vi "Alpha Ver 2.1.vi"() -> ()   [LabVIEW 2015]
uses:
  <instrlib>/Keithley 622x LV 2009/Utility/Typedefs/KE622x -- Instrument Type.ctl
  <instrlib>/Keithley 622x LV 2009/Keithley 622x.lvlib
panel:
  out "Measurements":string
  in  "Comments":string
  out "FILE":refnum<file>
  in  "Folder \nPrename":string
  out "Output command string":string
  out "Example of commands":string="*RST\nSOUR:PDEL:HIGH 1e-3\nSOUR:PDEL:LOW 0\nSOUR:PDEL:WIDT 500e-6\nSOUR:PDEL:SDEL 100e-6\nSOUR:PDEL:COUN INF\nSOUR:PDEL:RANG BEST\nSOUR:PDEL:INT 5\nSOUR:PDEL:LME 2\nTRAC:POIN 200\nSOUR:PDEL:ARM\nINIT:IMM"
  out "LM_com":string
  out "I_com":string
  out "R_com":string
  out "C_com":string
  out "SD_com":string
  out "W_com":string
  out "LL_com":string
  out "HL_com":string
  in  "INF Button":bool
  in  "prefix 2":u16(ring)
  in  "prefix":u16(ring)
  in  "Low Measure":u16(ring)=1 items=["1", "2"]
  in  "Interval":dbl=5.0 min=5.0 max=999999.0 step=1.0
  in  "Ranging":string(combo)="BEST"
  in  "Count":dbl=1.0 min=1.0 max=65536.0 step=1.0
  in  "Source Delay":dbl
  in  "Width":dbl
  in  "Low Level":dbl min=-0.105 max=0.105
  in  "High Level":dbl
  out "2182A \nconnected ?":string
  in  "STOP":bool
  out "Measurement\nUnits":string
  out "2182A Voltage \nRange":string
  out "error out":errorcluster
  # "Pulse Measurement System"
  # "SYSTEM INFORMATION"
  # "FILE CONFIGURATION"
  # "PULSE SETTINGS"
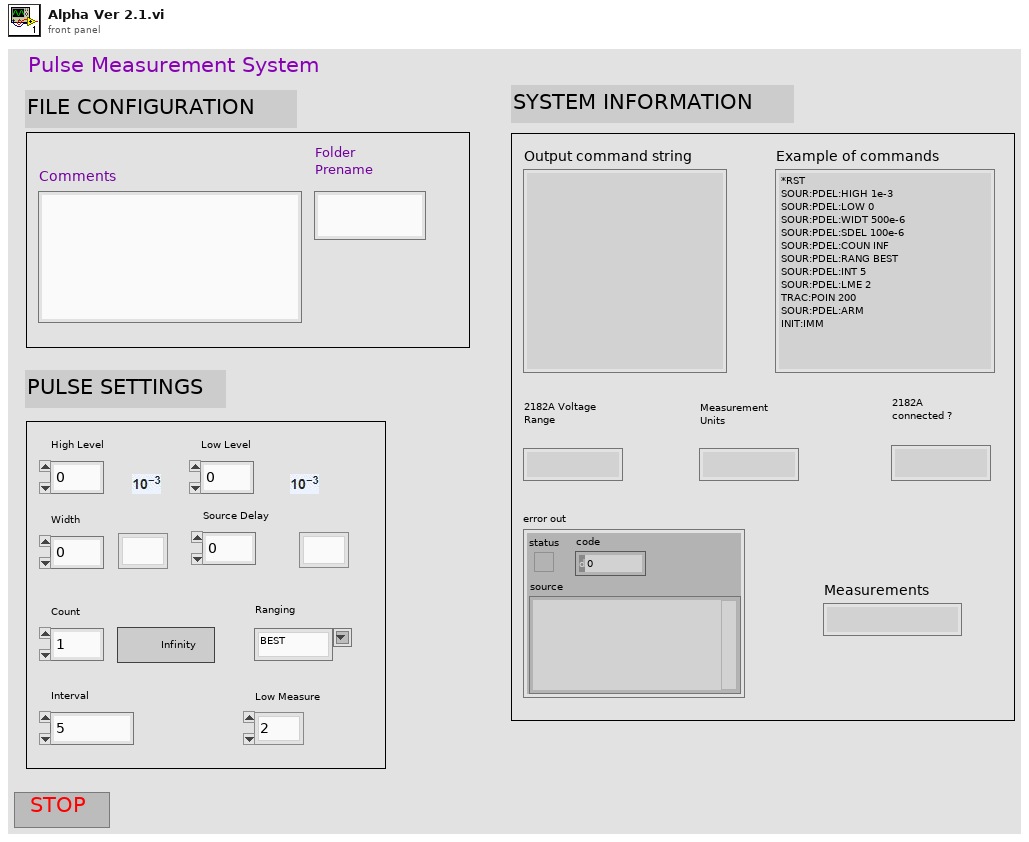
[diagram p1: front panel]
types:
  T1 = typedef "Keithley 622x.lvlib/KE622x -- Instrument Type.ctl" = enum16{"KE6220", "KE6221"}
  T2 = cluster{"VISA resource name out":refnum<visa-resource-name>, "error out":errorcluster}
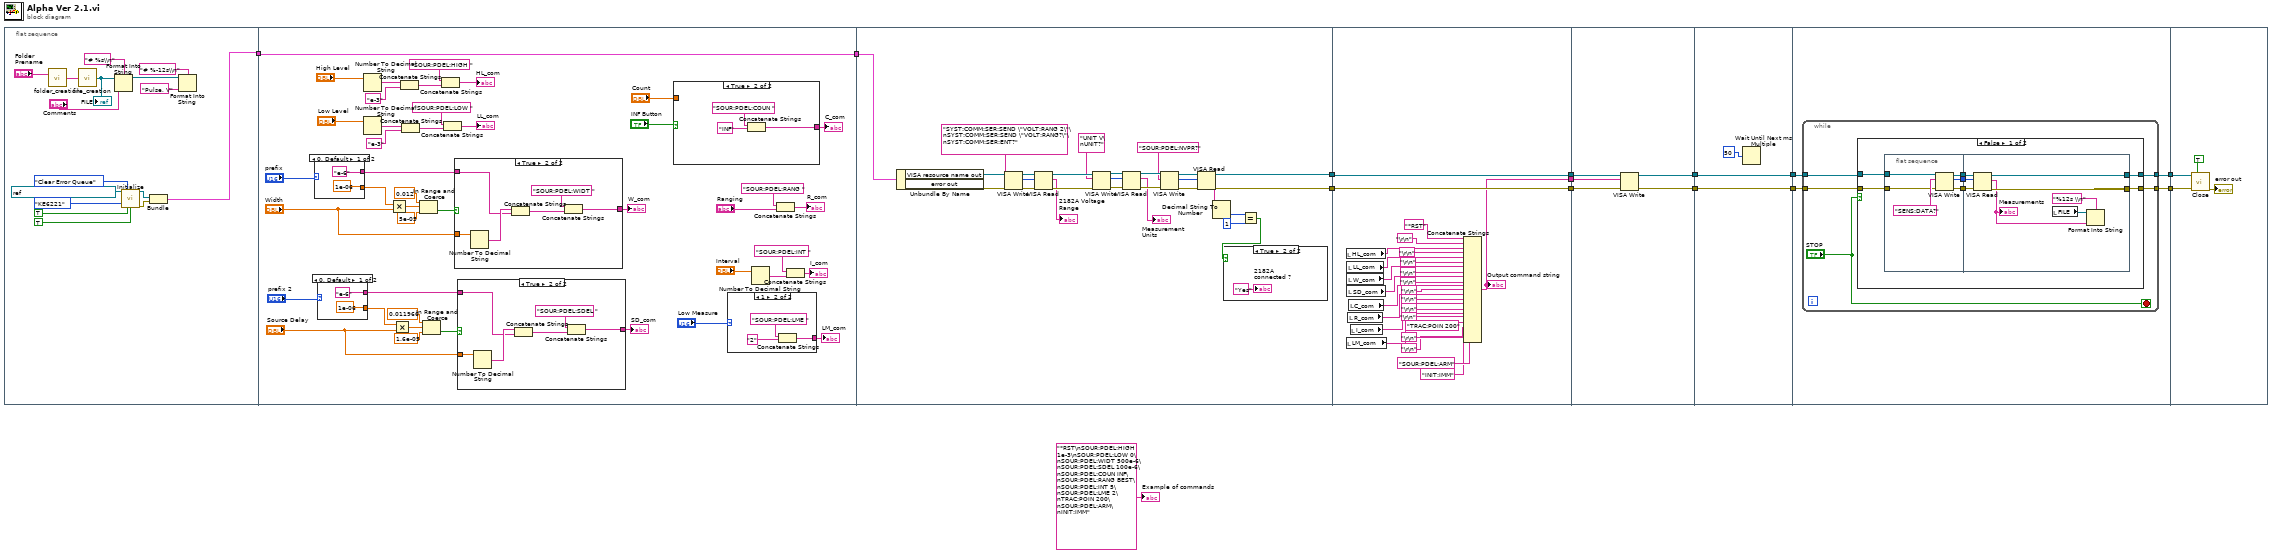
[diagram p0: block diagram]
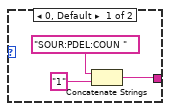
[diagram p2: hidden frame]
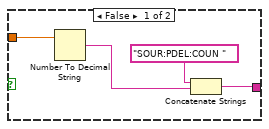
[diagram p3: hidden frame]
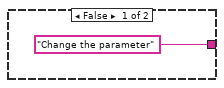
[diagram p4: hidden frame]
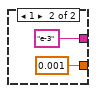
[diagram p5: hidden frame]
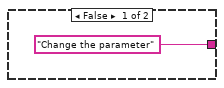
[diagram p6: hidden frame]
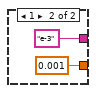
[diagram p7: hidden frame]
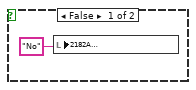
[diagram p8: hidden frame]
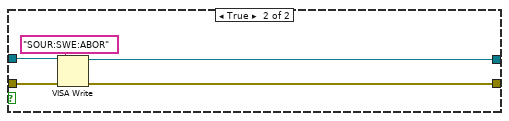
[diagram p9: hidden frame]
diagram:
  n1 = flat-sequence {
    tunnel: [w23] -> w12
    tunnel: w12 -> [w31]
    tunnel: [w31] -> w11
    tunnel: [w113] -> w10
    tunnel: [w112] -> w8
    tunnel: w11 -> [w111]
    tunnel: w10 -> [w163]
    tunnel: [w163] -> w9
    tunnel: w8 -> [w162]
    tunnel: [w162] -> w7
    tunnel: [w142] -> w5
    tunnel: w9 -> [w168]
    tunnel: [w167] -> w4
    tunnel: w7 -> [w166]
    tunnel: [w165] -> w2
    tunnel: w5 -> [w164]
    tunnel: w4 -> [w171]
    tunnel: [w171] -> w3
    tunnel: w2 -> [w170]
    tunnel: [w170] -> w1
    tunnel: w3 -> [w175]
    tunnel: w1 -> [w174]
    tunnel: [w173] -> w14
    tunnel: [w172] -> w13
    tunnel: w14 -> [w208]
    tunnel: w13 -> [w207]
    frame #0 {
      n2 = call "folder_creation.vi"("Name"="Folder \nPrename") -> ("String"=w21:string)
      n3 = call "file_creation.vi"("String"=w21) -> ("refnum out"=w20:refnum<file>)
      "FILE" <- w20
      n4 = Format Into String(format string="# %s\\n", initial string=w20, "Comments") -> (resulting string=w15:refnum<file>)  [unwired: 1 in, 1 out]
      n5 = call <instrlib>:"Initialize.vi"("VISA resource name"=refnum<visa-resource-name> "DC_AC_Current_Source_6221", "Error Queue Option"=enum16{"Clear Error Queue", "Error Query"}."Clear Error Queue", "Instrument Type"=KE622x_--_Instrument_Type."KE6221", "ID Query? (T)"=TRUE, "Reset? (T)"=TRUE) -> ("VISA resource name out"=w25:refnum<visa-resource-name>, "error out"=w24:errorcluster)  [unwired: 9 in]
      n6 = Bundle("VISA resource name out"=w25, "error out"=w24) -> (w23:T2)  [unwired: 1 in]
      n7 = Format Into String(format string="# %-12s\\n", initial string=w15, "Pulse, V" ("input 3")) -> ()  [unwired: 1 in, 2 out]
    }
    frame #1 {
      n8 = case shown="0, Default" "prefix" {
        tunnel: [1e-06 0.001] -> w54
        tunnel: ["e-6" ("string") "e-3" ("string")] -> w59
        frame 0, Default {
        }
        frame 1 {
        }
      }
      n9 = case shown="0, Default" "prefix 2" {
        tunnel: [1e-06 0.001] -> w49
        tunnel: ["e-6" ("string") "e-3" ("string")] -> w44
        frame 0, Default {
        }
        frame 1 {
        }
      }
      n10 = Number To Decimal String(number="High Level") -> (decimal integer string=w70:string)  [unwired: 1 in]
      n11 = Number To Decimal String(number="Low Level") -> (decimal integer string=w65:string)  [unwired: 1 in]
      n12 = Multiply(x=w54, y="Width") -> (x*y=w55:dbl)
      n13 = Multiply(x=w49, y="Source Delay") -> (x*y=w48:dbl)
      n14 = Concatenate Strings(w70, "e-3" ("string")) -> (w73:string)
      n15 = Concatenate Strings(w65, "e-3" ("string")) -> (w67:string)
      n16 = In Range and Coerce(upper limit=0.012, x=w55, lower limit=5e-05) -> (In Range?=w58:bool)  [unwired: 1 out]
      n17 = In Range and Coerce(upper limit=0.011966, x=w48, lower limit=1.6e-05) -> (In Range?=w45:bool)  [unwired: 1 out]
      n18 = Concatenate Strings("SOUR:PDEL:HIGH " ("string"), w73) -> (→"HL_com":string)
      n19 = Concatenate Strings("SOUR:PDEL:LOW " ("string"), w67) -> (→"LL_com":string)
      n20 = case shown="True" w58 {
        tunnel: w59 -> [_ w102]
        tunnel: "Width" -> [_ w104]
        tunnel: ["Change the parameter" w99] -> w61
        frame False {
        }
        frame True {
          n21 = Number To Decimal String(number=w104) -> (decimal integer string=w103:string)  [unwired: 1 in]
          n22 = Concatenate Strings(w103, w102) -> (w100:string)
          n23 = Concatenate Strings("SOUR:PDEL:WIDT " ("string"), w100) -> (w99:string)
        }
      }
      "W_com" <- w61
      n24 = case shown="True" w45 {
        tunnel: w44 -> [_ w91]
        tunnel: "Source Delay" -> [_ w93]
        tunnel: ["Change the parameter" w88] -> w52
        frame False {
        }
        frame True {
          n25 = Number To Decimal String(number=w93) -> (decimal integer string=w92:string)  [unwired: 1 in]
          n26 = Concatenate Strings(w92, w91) -> (w89:string)
          n27 = Concatenate Strings("SOUR:PDEL:SDEL " ("string"), w89) -> (w88:string)
        }
      }
      "SD_com" <- w52
      n28 = case shown="True" "INF Button" {
        tunnel: "Count" -> [w83 _]
        tunnel: [w81 w84] -> w43
        frame False {
          n29 = Number To Decimal String(number=w83) -> (decimal integer string=w80:string)  [unwired: 1 in]
          n30 = Concatenate Strings("SOUR:PDEL:COUN " ("string"), w80) -> (w81:string)
        }
        frame True {
          n31 = Concatenate Strings("SOUR:PDEL:COUN " ("string"), "INF") -> (w84:string)
        }
      }
      "C_com" <- w43
      n32 = case shown="1" "Low Measure" {
        tunnel: [w75 w77] -> w33
        frame 0, Default {
          n33 = Concatenate Strings("SOUR:PDEL:COUN " ("string"), "1" ("string")) -> (w75:string)
        }
        frame 1 {
          n34 = Concatenate Strings("SOUR:PDEL:LME " ("string"), "2") -> (w77:string)
        }
      }
      "LM_com" <- w33
      n35 = Number To Decimal String(number="Interval") -> (decimal integer string=w37:string)  [unwired: 1 in]
      n36 = Concatenate Strings("SOUR:PDEL:RANG " ("string"), "Ranging") -> (→"R_com":string)
      n37 = Concatenate Strings("SOUR:PDEL:INT " ("string"), w37) -> (→"I_com":string)
    }
    frame #2 {
      n38 = Unbundle By Name(w111) -> ("VISA resource name out"=w110:refnum<visa-resource-name>, "error out"=w109:errorcluster)
      n39 = VISA Write(VISA resource name=w110, write buffer="SYST:COMM:SER:SEND \"VOLT:RANG 2\"\nSYST:COMM:SER:SEND \"VOLT:RANG?\"\nSYST:COMM:SER:ENT?", error in (no error)=w109) -> (VISA resource name out=w133:refnum<visa-resource-name>, return count=w134:u32, error out=w132:errorcluster)
      n40 = VISA Read(VISA resource name=w133, byte count=w134, error in (no error)=w132) -> (VISA resource name out=w129:refnum<visa-resource-name>, read buffer=→"2182A Voltage \nRange":string, error out=w131:errorcluster)  [unwired: 1 out]
      n41 = VISA Write(VISA resource name=w129, write buffer="UNIT V\nUNIT?", error in (no error)=w131) -> (VISA resource name out=w125:refnum<visa-resource-name>, return count=w126:u32, error out=w127:errorcluster)
      n42 = VISA Read(VISA resource name=w125, byte count=w126, error in (no error)=w127) -> (VISA resource name out=w122:refnum<visa-resource-name>, read buffer=→"Measurement\nUnits":string, error out=w124:errorcluster)  [unwired: 1 out]
      n43 = VISA Write(VISA resource name=w122, write buffer="SOUR:PDEL:NVPR?", error in (no error)=w124) -> (VISA resource name out=w118:refnum<visa-resource-name>, return count=w119:u32, error out=w120:errorcluster)
      n44 = VISA Read(VISA resource name=w118, byte count=w119, error in (no error)=w120) -> (VISA resource name out=w113:refnum<visa-resource-name>, read buffer=w116:string, error out=w112:errorcluster)  [unwired: 1 out]
      n45 = Decimal String To Number(string=w116) -> (number=w115:i32)  [unwired: 2 in, 1 out]
      n46 = Equal?(x=w115, y=1) -> (x = y?=w117:bool)
      n47 = case shown="True" w117 {
        frame False {
          n48 = local write "2182A \nconnected ?"("No" ("2182A \nconnected ?")) -> ()
        }
        frame True {
          "2182A \nconnected ?" <- "Yes" ("2182A \nconnected ?")
        }
      }
    }
    frame #3 {
      n49 = local read "HL_com"() -> (w159:string)
      n50 = local read "LM_com"() -> (w145:string)
      n51 = local read "LL_com"() -> (w157:string)
      n52 = local read "W_com"() -> (w155:string)
      n53 = local read "SD_com"() -> (w153:string)
      n54 = local read "R_com"() -> (w150:string)
      n55 = local read "C_com"() -> (w151:string)
      n56 = local read "I_com"() -> (w147:string)
      n57 = Concatenate Strings("*RST" ("string"), "\r\n", w159, "\r\n", w157, "\r\n", w155, "\r\n", w153, "\r\n", w151, "\r\n", w150, "\r\n", w147, "\r\n", w145, "\r\n", "TRAC:POIN 200" ("string"), "\r\n", "SOUR:PDEL:ARM" ("string"), "\r\n", "INIT:IMM" ("string")) -> (w142:string)
      "Output command string" <- w142
    }
    frame #4 {
      n58 = VISA Write(VISA resource name=w168, write buffer=w164, error in (no error)=w166) -> (VISA resource name out=w167:refnum<visa-resource-name>, error out=w165:errorcluster)  [unwired: 1 out]
    }
    frame #5 {
      n59 = Wait Until Next ms Multiple(millisecond multiple=u32 50) -> ()  [unwired: 1 out]
    }
    frame #6 {
      n60 = while {
        tunnel: w175 -> [w180]
        tunnel: w174 -> [w179]
        tunnel: [w177] -> w173
        tunnel: [w176] -> w172
        stop <- "STOP" stop-if-true
        n61 = case shown="False" "STOP" {
          tunnel: w180 -> [w187 w205]
          tunnel: w179 -> [w186 w204]
          tunnel: [w181 w203] -> w177
          tunnel: [w182 w202] -> w176
          frame False {
            n62 = flat-sequence {
              tunnel: w187 -> [w192]
              tunnel: w186 -> [w191]
              tunnel: [w190] -> w185
              tunnel: [w189] -> w184
              tunnel: [w188] -> w183
              tunnel: w185 -> [w201]
              tunnel: w184 -> [w200]
              tunnel: w183 -> [w199]
              tunnel: [w198] -> w182
              tunnel: [w197] -> w181
              frame #0 {
                n63 = VISA Write(VISA resource name=w192, write buffer="SENS:DATA?", error in (no error)=w191) -> (VISA resource name out=w190:refnum<visa-resource-name>, return count=w188:u32, error out=w189:errorcluster)
              }
              frame #1 {
                n64 = VISA Read(VISA resource name=w201, byte count=w199, error in (no error)=w200) -> (VISA resource name out=w197:refnum<visa-resource-name>, read buffer=w195:string, error out=w198:errorcluster)  [unwired: 1 out]
                "Measurements" <- w195
                n65 = local read "FILE"() -> (w194:refnum<file>)
                n66 = Format Into String(format string="%12s \\n", initial string=w194, w195) -> ()  [unwired: 1 in, 2 out]
              }
            }
          }
          frame True {
            n67 = VISA Write(VISA resource name=w205, write buffer="SOUR:SWE:ABOR", error in (no error)=w204) -> (VISA resource name out=w203:refnum<visa-resource-name>, error out=w202:errorcluster)  [unwired: 1 out]
          }
        }
      }
    }
    frame #7 {
      n68 = call <instrlib>:"Close.vi"("VISA resource name"=w208, "Query For SCPI Errors? (T)"=TRUE, "error in (no error)"=w207) -> ("error out"=→"error out":errorcluster)  [unwired: 12 in]
    }
  }
  "Example of commands" <- "*RST\nSOUR:PDEL:HIGH 1e-3\nSOUR:PDEL:LOW 0\nSOUR:PDEL:WIDT 500e-6\nSOUR:PDEL:SDEL 100e-6\nSOUR:PDEL:COUN INF\nSOUR:PDEL:RANG BEST\nSOUR:PDEL:INT 5\nSOUR:PDEL:LME 2\nTRAC:POIN 200\nSOUR:PDEL:ARM\nINIT:IMM" ("write buffer")
